vi "Set Out.vi"(8 "error in":errorcluster, 11 "ProXR_IO in":refnum<class "ProXR.lvclass">) -> (0 "error out":errorcluster, 3 "ProXR_IO out":refnum<class "ProXR.lvclass">)   [LabVIEW 2019, in "ProXR.lvlib" / "ProXR.lvclass"]
uses:
  Library/ProXR.lvclass
  C:/Users/Public/Documents/Development/builds/Instruments/DIG_IO.lvlibp/Library/DIG_IO.lvclass
  builds/Instruments/DIG_IO.lvlibp/Accessors/Read ToggleTarget.vi
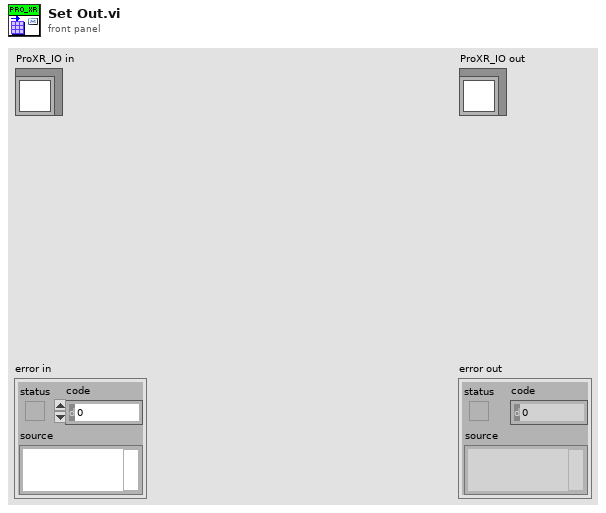
[diagram p1: front panel]
types:
  T1 = cluster{"Position":u32, "Bank":u32, "Value":bool}
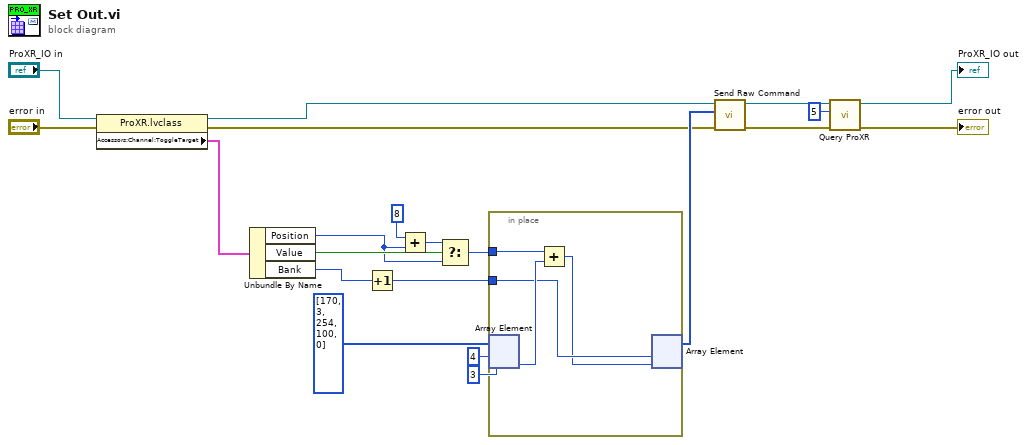
[diagram p0: block diagram]
diagram:
  n1 = property class="ProXR.lvclass"(reference="ProXR_IO in", error in="error in") -> (reference out=w12:refnum<class "ProXR.lvclass">, error out=w11:errorcluster, "Accessors:Channel:ToggleTarget"=w4:T1)
  n2 = Unbundle By Name(w4) -> ("Position"=w2:u32, "Value"=w3:bool, "Bank"=w1:u32)
  n3 = Increment(x=w1) -> (x+1=w10:u32)
  n4 = Add(x=u8 8, y=w2) -> (x+y=w21:u32)
  n5 = Select(t=w21, s=w3, f=w2) -> (s? t:f=w19:u32)
  n6 = in-place {
    in-place-border: w19 -> [w25]
    in-place-border: w10 -> [w23]
    n7 = in-place-array #1(u8[] [170, 3, 254, 100, 0], 4, 3) -> (w24:u8)  [unwired: 1 out]
    n8 = Add(x=w25, y=w24) -> (x+y=w22:u32)
    n9 = in-place-array #1(w23, w22) -> (w18:u8[])  [unwired: 2 out]
  }
  n10 = call "Send Raw Command.vi"("error in"=w11, "Raw Command"=w18, "ProXR_IO in"=w12) -> ("error out"=w8:errorcluster, "ProXR_IO out"=w9:refnum<class "ProXR.lvclass">)  [unwired: 7 in]
  n11 = call "Query ProXR.vi"("error in"=w8, "Bytes to Read"=u32 5, "ProXR_IO in"=w9) -> ("error out"=→"error out":errorcluster, "ProXR_IO out"=→"ProXR_IO out":refnum<class "ProXR.lvclass">)  [unwired: 6 in, 1 out]
